vi "Servo(m) (subVI).vi"(0 "PWM channel 2":tag="B/PWM0", 3 "error in (no error)":errorcluster) -> (10 "error out":errorcluster)   [LabVIEW 2017]
uses:
  <vilib>/myRIO/Instrument Drivers/Onboard IO/PWM/typedefs/PWM Reference.ctl
  <vilib>/myRIO/Common/Instrument Driver Framework/Utilities/typedefs/myRIO Generic Hardware Reference.ctl
  <vilib>/myRIO/Common/Instrument Driver Framework/Utilities/typedefs/Hardware Version Enum.ctl
  <vilib>/myRIO/Common/Instrument Driver Framework/Utilities/typedefs/myRIO v1.0 Reference.ctl
  <vilib>/myRIO/Common/Instrument Driver Framework/Utilities/typedefs/Generic FPGA Reference.ctl
  <vilib>/myRIO/Common/Instrument Driver Framework/myRIO v1.0/PWM/typedefs/PWM Channels Enum.ctl
  <vilib>/myRIO/Instrument Drivers/Onboard IO/PWM/typedefs/PWM Configuration.ctl
  <vilib>/Utility/error.llb/Error Cluster From Error Code.vi
  <vilib>/myRIO/Instrument Drivers/Onboard IO/PWM/PWM.lvlib
panel:
  in  "duty cycle [%]":dbl=50.0
  out "PWM Ref Out":T1
  in  "Stop Button":bool
  in  "freq [Hz]":dbl=50.0
  # "Servo"
  # "Big servo: 506 - 0 deg"
  # "533 - 90 deg"
  # "Small servo: 620 - 0 deg"
  # "990 - 90 deg"
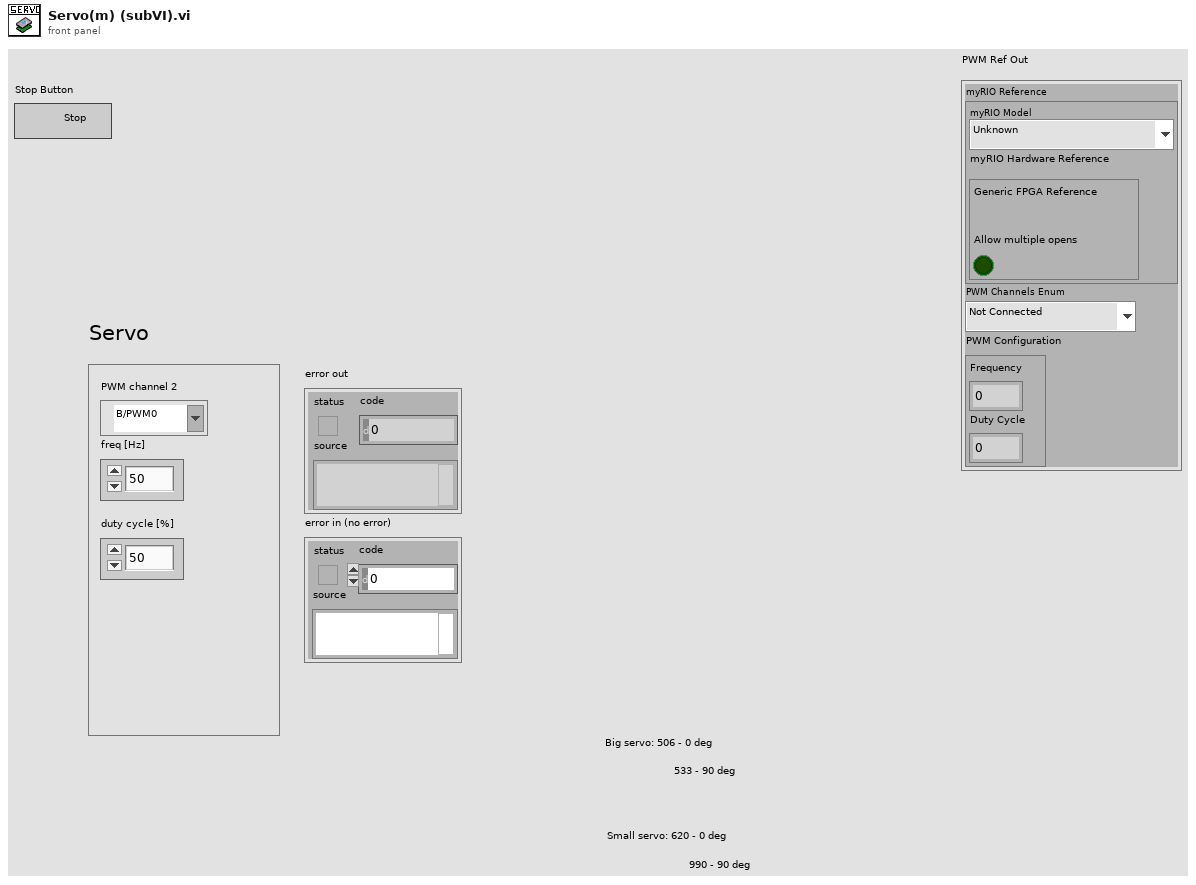
[diagram p1: front panel]
types:
  T1 = typedef "PWM.lvlib/PWM Reference.ctl" = cluster{"myRIO Reference":T2, "PWM Channels Enum":T6, "PWM Configuration":T7}
  T2 = typedef "myRIO Generic Hardware Reference.ctl" = cluster{"myRIO Model":T3, "myRIO Hardware Reference":T4}
  T3 = typedef "Hardware Version Enum.ctl" = enum16{"Unknown", "myRIO-1900", "myRIO-1950", "roboRIO", "NI ELVIS RIO CM"}
  T4 = typedef "myRIO v1.0 Reference.ctl" = cluster{"Generic FPGA Reference":T5, "Allow multiple opens":bool}
  T5 = typedef "Generic FPGA Reference.ctl" = refnum<k20>
  T6 = typedef "PWM Channels Enum.ctl" = enum16{"Not Connected", "C/PWM0", "C/PWM1", "A/PWM0", "A/PWM1", "A/PWM2", "B/PWM0", "B/PWM1", "B/PWM2", "PWM/PWM0", "PWM/PWM1", "PWM/PWM2", "PWM/PWM3", "PWM/PWM4", "PWM/PWM5", "PWM/PWM6", "PWM/PWM7", "PWM/PWM8", "PWM/PWM9"}
  T7 = typedef "PWM.lvlib/PWM Configuration.ctl" = cluster{"Frequency":dbl, "Duty Cycle":dbl}
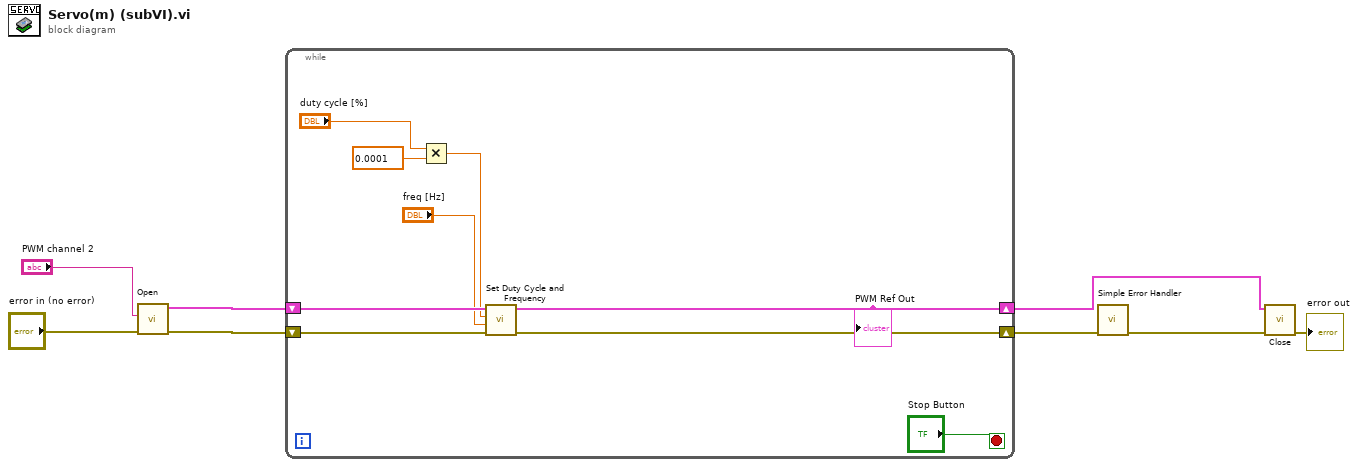
[diagram p0: block diagram]
diagram:
  n1 = call <vilib>:"Open.vi"("error in (no error)"="error in (no error)", "Channel Name"="PWM channel 2") -> ("error out"=w2:errorcluster, "PWM Ref Out"=w1:T1)  [unwired: 8 in]
  n2 = while {
    shift-right: [w16] -> w5
    shift-left: w2 -> [w15]
    shift-right: [w17] -> w6
    shift-left: w1 -> [w14]
    stop <- "Stop Button" stop-if-true
    n3 = Multiply(x="duty cycle [%]", y=0.0001) -> (x*y=w12:dbl)
    n4 = call <vilib>:"Set Duty Cycle and Frequency.vi"("error in (no error)"=w15, "Frequency [Hz]"="freq [Hz]", "Duty Cycle"=w12, "PWM Ref In"=w14) -> ("error out"=w16:errorcluster, "PWM Ref Out"=w17:T1)  [unwired: 5 in]
    "PWM Ref Out" <- w17
  }
  n5 = call <vilib>:"Simple Error Handler.vi"("error in (no error)"=w5) -> ("error out"=w8:errorcluster)  [unwired: 4 in, 4 out]
  n6 = call <vilib>:"Close.vi"("error in (no error)"=w8, "PWM Ref In"=w6) -> ("error out"=→"error out":errorcluster)  [unwired: 9 in]
